vi "qONT.vi"(0 "System no.":i32=1 min=1 max=4 step=1, 2 "Axes to query":string[](array[string]), 3 "All axes?":bool, 4 "Axis identifier?":bool=TRUE, 5 "error in":errorcluster) -> (14 "Axis on target?":bool[](array[boolean]), 19 "error out":errorcluster)   [LabVIEW 2026]
doc: "GCS 3.0\n=====\n\nONT? (Get On-Target State)\n\nDescription \nQueries the on-target state of the axes.\n\nFormat\nONT?[ <AxisID>]\n\nArguments\nONT? without arguments queries all axes of the controller.\n<AxisID>\nAn axis of the controller\nThe available axes can be queried with USG? SYS.\nPossible values: Alias of the axis (p. 94) \n\nResponse\n{<AxisID>\"=\"<OnTargetState>LF}\n<OnTargetState>\nOn-target state of the axis\nFor the criteria for determining the on-target state, see \"Notes\".\nPossible values:\n1 = Axis on target\n0 = Axis not on target\n\nNotes\nIt is always possible to determine the on-target state. However, the on-target state can only \nhave the value 1 in a closed-loop mode of operation. For further details on the modes of \noperation, see \"Drive State Machine\" (p. 101). \nThe controller determines the on-target state based on the following criteria:\n- Settling window around the target value (specified by the parameter AXIS_n CNTR_n \n0x111 Settle Window)\n- Delay time for setting the on-target state (specified by the parameter AXIS_n CNTR_n \n0x112 Settle Time)\nThe on-target state has the value 1 when the profile generator has finished outputting the \ndynamics profile and the following is valid:\n- The current value of the control variable is inside the settling window and stays there at \nleast for the duration of the delay time.\n- If the value for the delay time is set to 0: The current value of the control variable is in\nthe settling window.\nWhen a new target value is set, the on-target state is reset to zero.\nThe on-target state is also displayed in the status register of the axis (p. 97), which can be \nqueried with the STV? command (p. 66). \n\nUser command level\nUSR\n\n\nGCS 2.0\n=====\n\nIndicates whether or not queried axis is at target position.\n\nE-755: If All axes? = TRUE, then Axis identifier? can be FALSE. Command not available for E-755.101 \nE-816: All axes? = FALSE, only one axis per command allowed.\nAll other systems: If All axes? = TRUE, then Axis identifier? can be FALSE."
panel:
  # "ONT? (Get On-Target State)\n\nQueries the on-target state of the axes."
  # "Query"
  # "If all axes: use"
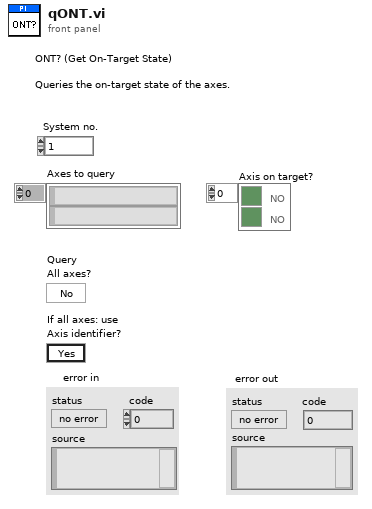
[diagram p1: front panel]
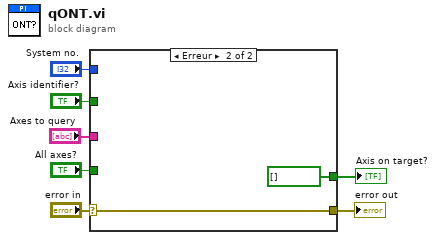
[diagram p0: block diagram]
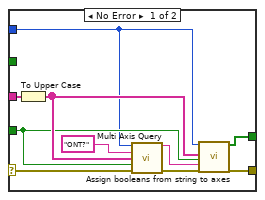
[diagram p2: hidden frame]
diagram:
  n1 = case shown="Erreur" "error in" {
    selector: "error in" -> [w16 w19]
    tunnel: [w11 bool[] [] ("Booleans")] -> w2
    tunnel: "Axes to query" -> [w17 _]
    tunnel: [w13 w19] -> w3
    tunnel: "System no." -> [w8 _]
    tunnel: "All axes?" -> [w9 _]
    tunnel: "Axis identifier?" -> [_ _]
    frame No Error {
      n2 = To Upper Case(1:w17) -> (0:w12:string[])
      n3 = call "Multi Axis Query.vi"("System no."=w8, "Command"="ONT?", "Axis"=w12, "All axes?"=w9, "error in (no error)"=w16) -> ("Answer"=w10:string, "error out"=w14:errorcluster)  [unwired: 9 in]
      n4 = call "Assign booleans from string to axes.vi"("System no."=w8, "Queried axes"=w12, "All axes queried?"=w9, "Input String"=w10, "error in"=w14) -> ("Booleans"=w11:bool[], "error out"=w13:errorcluster)  [unwired: 13 in]
    }
    frame Error {
      (unwired) string[] [] ("Axes to query out")
    }
  }
  "error out" <- w3
  "Axis on target?" <- w2
